vi "GetType.vi"(0 "reference in":refnum<class "Proccess.lvclass">) -> (4 "reference out":refnum<class "Proccess.lvclass">, 6 "obj_type":T1)   [LabVIEW 2019, in "Proccess.lvclass"]
uses:
  Proccess.lvclass
  Logger_class/ObjType.ctl
  Logger_class/Logger.lvclass
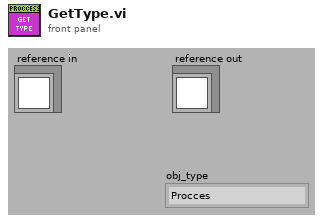
[diagram p1: front panel]
types:
  T1 = typedef "Logger.lvclass/ObjType.ctl" = enum16{"Procces", "Device", "SignalA", "SignalD", "DI", "DO", "DA", "AI", "AO", "AA", "GUI"}
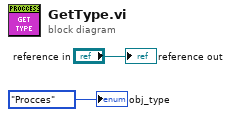
[diagram p0: block diagram]
diagram:
  "reference out" <- "reference in"
  "obj_type" <- ObjType."Procces" ("obj_type")
